vi "Insight_RW_SweepRate.vi"(7 "Parameter Type":enum16{"Value", "MAXimum", "MINimum", "DEFault"}(ring), 8 "error in (no error)":errorcluster, 9 "Mode (Read / Write)":enum8{"Write", "Read"}(ring), 10 "Sweep Rate (kHz)":dbl=100.0 format="%.4g", 11 "telnet connection":T1) -> (0 "error out":errorcluster, 1 "response data":string, 2 "Sweep Rate (kHz)":dbl format="%.4g", 3 "telnet  connection out":T1)   [LabVIEW 2015]
doc: "Insight Photonic Solutions\n\nThis VI reads or writes the Sweep Rate of the laser.\n\nSweep Rate defined as the inverse of the time the laser is sweeping. Alternatively, this is the laser's clock rate divided by the number of sample points.\n\nThis VI is different that Insight_RW_RepetitionRate.vi, which reads or writes the Sweep Repetition Rate of the laser, i.e. how frequently the laser restarts a new sweep.\n\nINPUTS\n\nMode - Tells the VI whether the command is a Read or a Write. (Default = Read).\nParameter Type - Tells the VI whether the command should use a Value or a keyword MAXimum, MINimum or DEFault to set the parameter value. (Default = Value).\nSweep Rate (kHz) - The numeric value to set the Sweep Rate of a sweep. (Default = 100).\nerror in - The standard LabView Error cluster. Use this to enforce sequentiality and error tracking.\n\nOUTPUTS\n\nresponse data - the complete response string from the laser\nSweep Rate (kHz) - the Sweep Rate written to or read from the laser\nerror out - the standard error cluster. Reports errors in reading or writing to the laser, or passes through errors from before this VI.\n\nver 3.5 - original release, based on the VI Insight_RW_RepetitionRate.vi. This VI implements the new meaning of the command :CONFigure:SWEep:RATE. The re-definition of this command occurs in Atlas 3.5."
uses:
  Telnet Session.ctl
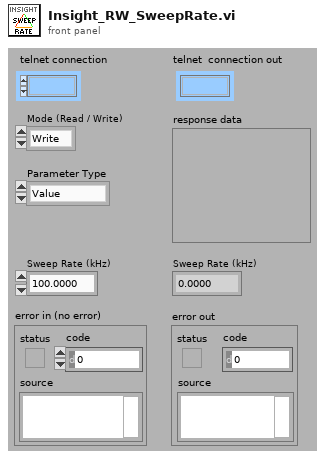
[diagram p1: front panel]
types:
  T1 = typedef "Telnet Session.ctl" = refnum<k1>
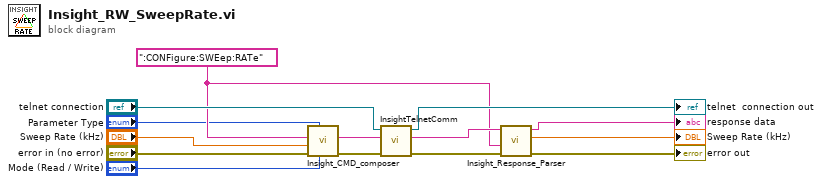
[diagram p0: block diagram]
diagram:
  w4 = ":CONFigure:SWEep:RATe" ("String")
  n1 = call "Insight_CMD_composer.vi"("Mode (Read / Write)"="Mode (Read / Write)", "Parameter Type"="Parameter Type", "error in (no error)"="error in (no error)", "Value"="Sweep Rate (kHz)", "CMD"=w4) -> ("error out"=w7:errorcluster, "Command String"=w5:string)  [unwired: 5 in]
  n2 = call "InsightTelnetComm.vi"("error in"=w7, "write buffer (\"\")"=w5, "telnet connection"="telnet connection") -> ("error out"=w12:errorcluster, "response data"=w8:string, "telnet  connection out"=→"telnet  connection out":T1)  [unwired: 4 in]
  n3 = call "Insight_Response_Parser.vi"("error in (no error)"=w12, "Command String"=w4, "Laser Response In"=w8) -> ("error out"=→"error out":errorcluster, "Value"=→"Sweep Rate (kHz)":dbl, "Laser Response Out"=→"response data":string)  [unwired: 6 in]
